vi "SubVI.vi"   [LabVIEW 2017]
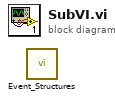
[diagram p0: block diagram]
diagram:
  n1 = call "Event_Structures.vi"() -> ()  [unwired: 1 in]
